vi "Parameter_Sweep_prep.vi"(8 "error in (no error)":errorcluster, 11 "Acquired z-plane index / volume index":i32) -> (0 "error out":errorcluster)   [LabVIEW 2020]
uses:
  Typedefs/fgv_actions.ctl
  Global Variables/gl_UI Ctrl Refs.vi
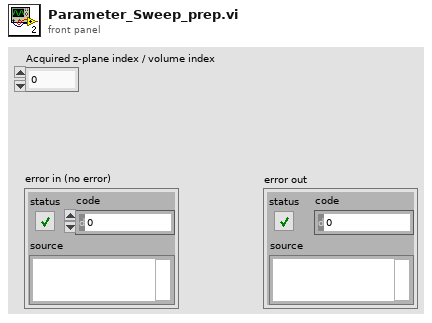
[diagram p1: front panel]
types:
  T1 = typedef "fgv_actions.ctl" = enum16{"Get", "Set"}
  T2 = typedef "UI ctrl refs cluster.ctl" = cluster{"Top level VI path":path, "Top level VI ref":refnum<vi>, "User menu ref":refnum<k9>, "Sub Panel control":refnum<vi>, "Imaging Param Tab":refnum<vi>, "Occurrence-Start drivers":refnum<k4>, "Occurrence-Speed logging initialised":refnum<k4>, "Occurrence-XYZ stage initialised":refnum<k4>, "Exit button":refnum<vi>, "Status ind":refnum<vi>, "Set as origin":refnum<vi>, "Speed Logging":refnum<vi>, "Time Lapse":refnum<vi>, "Live Imaging":refnum<vi>, "AOL Z Stack":refnum<vi>, "Motor Z Stack":refnum<vi>, "Funct Acq button":refnum<vi>, "Hard Shutter":refnum<vi>, "Virtual Shutter":refnum<vi>, "Laser Power":refnum<vi>, "AOL Mode":refnum<vi>, "Frame Size":refnum<vi>, "Field of View":refnum<vi>, "Dwell Time":refnum<vi>, "Zoom":refnum<vi>, "AOL Z":refnum<vi>, "Objective":refnum<vi>, "Axis":refnum<vi>, "Paths & Names":refnum<vi>, "Experiment folder path (ind.)":refnum<vi>, "Last State (Ind.)":refnum<vi>, "Averages":refnum<vi>, "Angle (degrees)":refnum<vi>, "X centre":refnum<vi>, "Y centre":refnum<vi>, "Plane Mode":refnum<vi>, "# Planes":refnum<vi>, "Z Start":refnum<vi>, "Z Stop":refnum<vi>, "Z Step":refnum<vi>, "PMT 1":refnum<vi>, "PMT 2":refnum<vi>, "Stage XYZ Position":refnum<vi>, "Pockels@Z Start":refnum<vi>, "Pockels@Z Stop":refnum<vi>, "Obtain Z Start":refnum<vi>, "Obtain Z Stop":refnum<vi>, "Live stim.trig.period":refnum<vi>, "Live stim.trig.enable":refnum<vi>, "Movement Correction":refnum<vi>, "Load Reference Image":refnum<vi>, "XY Stage Move":refnum<vi>, "MovCor Cluster":refnum<vi>, "RefDAQParam":refnum<vi>, "Funct. Acq. Pockels Modulation":refnum<vi>, "Ref Laser Power":refnum<vi>, "Enable Video Recording":refnum<vi>, "Video Record-Live Imaging":refnum<vi>, "Video Record-Funct acq":refnum<vi>, "Reference Source":refnum<vi>, "AOL Z-stack Chirps Ready (ind)":refnum<vi>, "Target time between mov.cor. ref triggers (ms)":refnum<vi>, "Funct. Acq. Ref frame save":refnum<vi>, "Tracking button":refnum<vi>, "Show ref plots window":refnum<vi>, "Center freq ind (nm)":refnum<vi>, "Pickup mode (ind)":refnum<vi>, "Logging queue (ind)":refnum<vi>, "Back aperture power (ind.)":refnum<vi>, "Power after objective (ind.)":refnum<vi>, "Switch user":refnum<vi>, "Ls1 Conn. Status":refnum<vi>, "Ls1Tuning Status":refnum<vi>, "Ls1 Faults":refnum<vi>, "Ls1 Connection":refnum<vi>, "Ls1 Mode":refnum<vi>, "Ls1 POWER [mW]":refnum<vi>, "Ls1Shutter":refnum<vi>, "Ls1 Wavelength":refnum<vi>, "Ls1 Note":refnum<vi>, "Ls1 Confirm Wav":refnum<vi>, "Ls1 PreChrp Prism1":refnum<vi>, "Ls1 PreChrp Prism2":refnum<vi>, "Ls1 wav top Ind":refnum<vi>, "Ls1 power top Ind":refnum<vi>, "Ls1 Pump peak Hold":refnum<vi>, "Ls1 Status Ind":refnum<vi>, "Ls1 wav cancel":refnum<vi>, "Experiment Type":refnum<vi>, "Biology Information":refnum<vi>, "Camera recording status":refnum<vi>, "Optimise Obj. Pos.":refnum<vi>}
  T3 = typedef "Parameter sweep modes.ctl" = enum16{"None Selected", "Multibeam Sep. [um]", "Dwell Time [us]"}
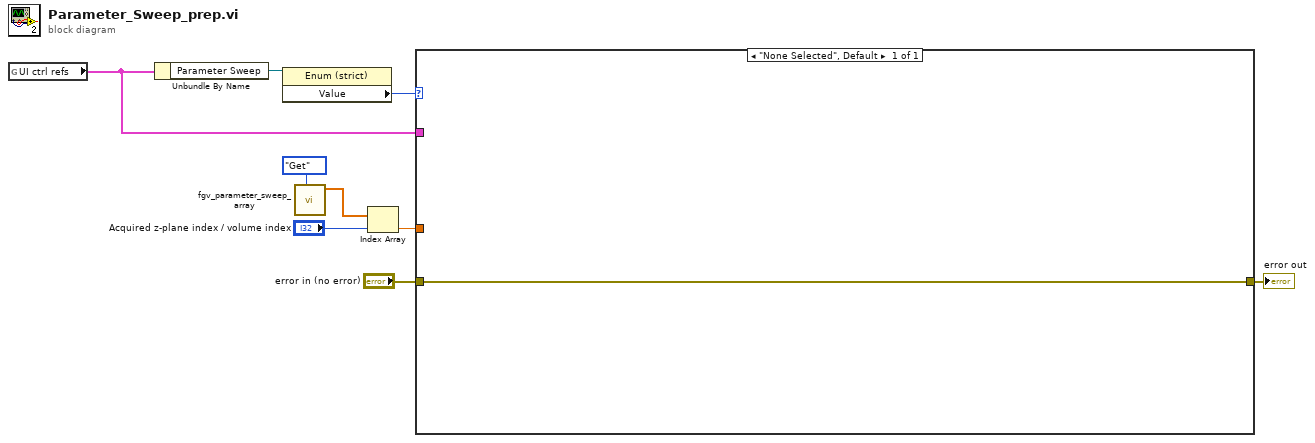
[diagram p0: block diagram]
diagram:
  n1 = global read "gl_UI Ctrl Refs.vi" "UI ctrl refs"() -> (w4:T2)
  n2 = Unbundle By Name(w4) -> ("Parameter Sweep"=w6:refnum<vi>)
  n3 = property class="Enum (strict)"(reference=w6) -> ("Value"=w5:T3)  [unwired: 1 in, 2 out]
  n4 = call "fgv_parameter_sweep_array.vi"("FGV Actions"=fgv_actions."Get") -> ("Sweep Parameter Array"=w7:dbl[])  [unwired: 8 in, 2 out]
  n5 = Index Array(array=w7, index="Acquired z-plane index / volume index") -> (element=w3:dbl)
  n6 = case shown="\"None Selected\", Default" w5 {
    tunnel: w4 -> [_]
    tunnel: w3 -> [_]
    tunnel: "error in (no error)" -> [w10]
    tunnel: [w10] -> w1
    frame "None Selected", Default {
    }
  }
  "error out" <- w1
